vi "Get_Previous_Value_Bool.vi"(1 "Input":bool) -> (0 "Output":bool)   [LabVIEW 2018, in "Tracker.lvlib"]
uses:
  Tracker.lvlib
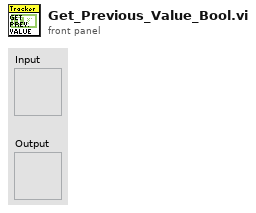
[diagram p1: front panel]
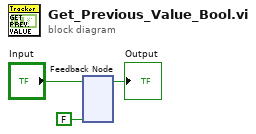
[diagram p0: block diagram]
diagram:
  n1 = feedback-in #1("Input") -> ()
  n2 = feedback #1(FALSE ("Input")) -> (→"Output":bool)
